vi "Loop.vi"() -> ()   [LabVIEW 2023]
panel:
  out "Index 2":i32
  out "Waveform Chart 2":dbl(graph)
  out "Waveform Chart":dbl(graph)
  in  "stop":bool
  out "Index":i32
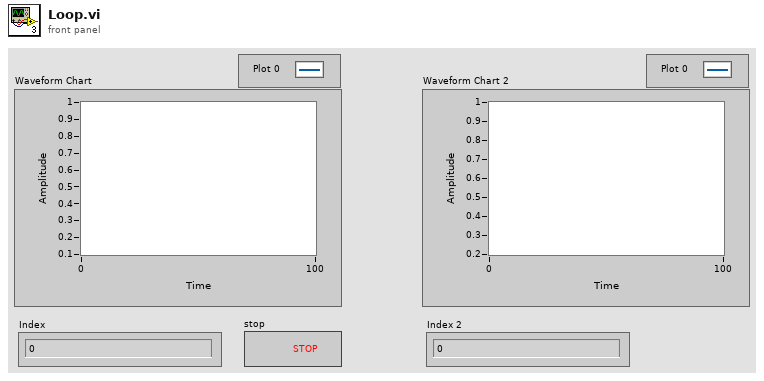
[diagram p1: front panel]
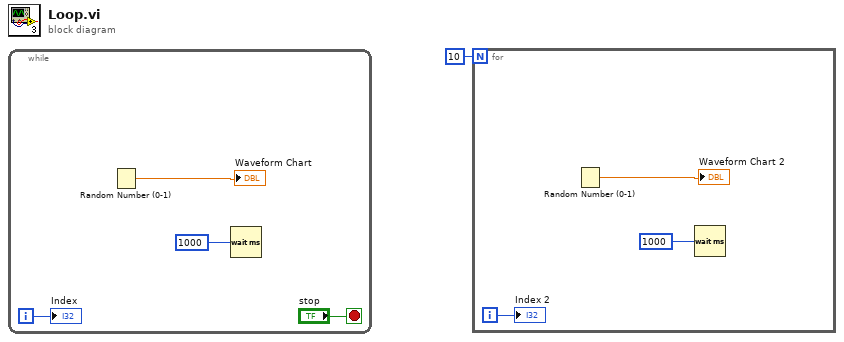
[diagram p0: block diagram]
diagram:
  n1 = while {
    i -> [w5]
    stop <- "stop" stop-if-true
    n2 = Random Number (0-1)() -> (number: 0 to 1=→"Waveform Chart":dbl)
    n3 = Wait (ms)(milliseconds to wait=u32 1000) -> ()  [unwired: 1 out]
    "Index" <- w5
  }
  n4 = for {
    N: 10 -> [_]
    i -> [w8]
    n5 = Random Number (0-1)() -> (number: 0 to 1=→"Waveform Chart 2":dbl)
    n6 = Wait (ms)(milliseconds to wait=u32 1000) -> ()  [unwired: 1 out]
    "Index 2" <- w8
  }
